vi "Configure.vi"(0 "VISA resource name":refnum<visa-resource-name>, 1 "Voltage(0 Volts)":dbl format="%.3f", 2 "Protection(None:0)":u16(ring) items=["None", "Overcurrent protection", "Overvoltage protection", "Overcurrent and overvoltage protection", "Clear overvoltage condition", "Clear overcurrent protection", "Set time delay"], 5 "Ouput(On:T)":bool=TRUE, 7 "Voltage Mode(F:Immediate)":bool, 9 "Current Mode(F:Immediate)":bool, 11 "error in (no error)":errorcluster, 12 "Current(0 Amps)":dbl format="%.3f", 13 "Overvoltage prot value(50 Volts)":dbl=50.0 format="%.3f", 14 "Time Delay(0 seconds)":dbl format="%.4f") -> (4 "VISA resource name out":refnum<visa-resource-name>, 15 "error out":errorcluster)   [LabVIEW 2012, in "Agilent 66XX Series.lvlib"]
doc: "This vi configures voltage, current, and overvoltage/current protection. It is also responsible for clearing any protection as well as determining whether the output on the power supply changes immediately or is triggered on the HP-IB bus. NOTE: In order to clear the overcurrent or overvoltage condition, the cause of the condition must be removed first. All values are shown in Volts and Amps."
uses:
  <instrlib>/Agilent 66XX Series/Agilent 66XX Series.lvlib
panel:
  # "On"
  # "Off"
  # "Trigger"
  # "Immediate"
  # "Trigger"
  # "Immediate"
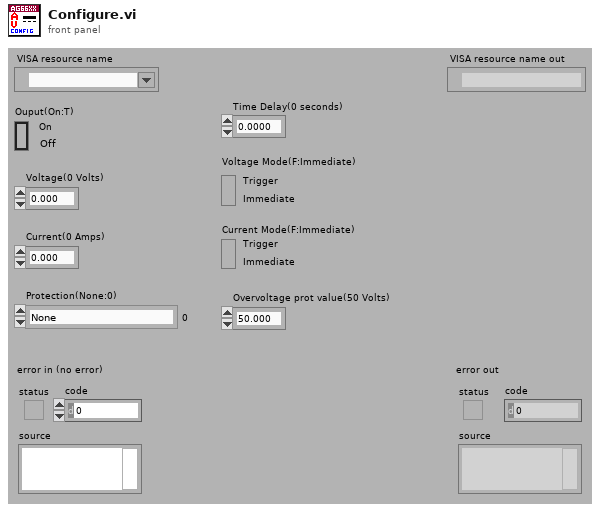
[diagram p1: front panel]
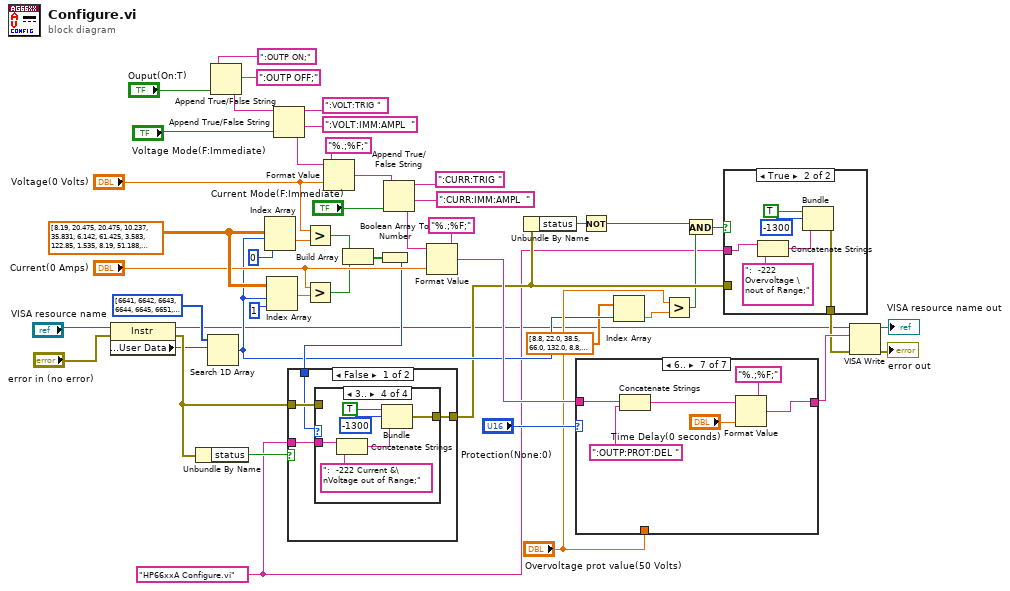
[diagram p0: block diagram]
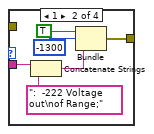
[diagram p4: hidden frame]
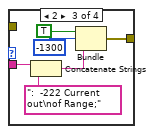
[diagram p5: hidden frame]
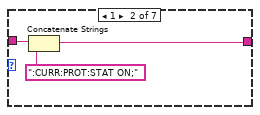
[diagram p8: hidden frame]
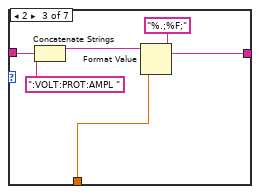
[diagram p9: hidden frame]
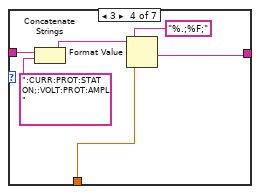
[diagram p10: hidden frame]
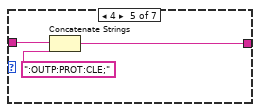
[diagram p11: hidden frame]
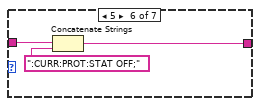
[diagram p12: hidden frame]
diagram:
  w30 = dbl[][] [[8.19, 20.475], [20.475, 10.237], [35.831, 6.142], [61.425, 3.583], [122.85, 1.535], [8.19, 51.188], [20.475, 25.594], [35.831, 15.356], [61.425, 9.214], [122.85, 4.095], [8.19, 225.23], [20.475, 102.37], [35.831, 61.43], [61.425, 35.83], [122.85, 18.43], [5.125, 895.0], [8.19, 592.0], [21.5, 246.0], [32.75, 164.0], [41.0, 131.0], [15.375, 450.0], [30.75, 225.0], [61.5, 112.0], [81.9, 30.71]] ("Range Values")
  w5 = "HP66xxA Configure.vi"
  n1 = property class="Instr"(reference="VISA resource name", error in="error in (no error)") -> (reference out=w4:refnum<visa-resource-name>, error out=w3:errorcluster, "General Settings:User Data"=w2:u32)
  n2 = Unbundle By Name(w3) -> ("status"=w34:bool)
  n3 = Search 1D Array(1D array=u32[] [6641, 6642, 6643, 6644, 6645, 6651, 6652, 6653, 6654, 6655, 6671, 6672, 6673, 6674, 6675, 6680, 6681, 6682, 6683, 6684, 6690, 6691, 6692, 4356] ("Number"), element=w2) -> (index of element=w18:i32)  [unwired: 1 in]
  n4 = Append True/False String(1:"Ouput(On:T)", 2:":OUTP OFF;", 3:":OUTP ON;") -> (0:w11:string)  [unwired: 1 in]
  n5 = Index Array(array=w30, index (row)=w18, index (col)=0) -> (element=w29:dbl)
  n6 = Index Array(array=w30, index (row)=w18, index (col)=1) -> (element=w27:dbl)
  n7 = Append True/False String(1:"Voltage Mode(F:Immediate)", 2:":VOLT:IMM:AMPL  ", 3:":VOLT:TRIG ", 4:w11) -> (0:w47:string)
  n8 = Greater?(x="Voltage(0 Volts)", y=w29) -> (0:w22:bool)
  n9 = Greater?(x="Current(0 Amps)", y=w27) -> (0:w21:bool)
  n10 = Format Value(string ("")=w47, format string="%.;%F;", value (0)="Voltage(0 Volts)") -> (output string=w41:string)
  n11 = Build Array(w22, w21) -> (w20:bool[])
  n12 = Boolean Array To Number(Boolean array=w20) -> (number=w19:u32)
  n13 = case shown="False" w34 {
    tunnel: [w53 w73] -> w10
    tunnel: w3 -> [w52 w73]
    tunnel: w5 -> [w51 _]
    tunnel: w19 -> [w50 _]
    frame False {
      n14 = case shown="3.." w50 {
        tunnel: [w54 w55 w61 w67] -> w53
        tunnel: w52 -> [w54 _ _ _]
        tunnel: w51 -> [_ w56 w62 w68]
        frame ..0 {
        }
        frame 1 {
          n15 = Concatenate Strings(w56, ":  -222 Voltage out\nof Range;") -> (w57:string)
          n16 = Bundle(TRUE, -1300, w57) -> (w55:errorcluster)  [unwired: 1 in]
        }
        frame 2 {
          n17 = Concatenate Strings(w62, ":  -222 Current out\nof Range;") -> (w63:string)
          n18 = Bundle(TRUE, -1300, w63) -> (w61:errorcluster)  [unwired: 1 in]
        }
        frame 3.. {
          n19 = Concatenate Strings(w68, ":  -222 Current &\nVoltage out of Range;") -> (w69:string)
          n20 = Bundle(TRUE, -1300, w69) -> (w67:errorcluster)  [unwired: 1 in]
        }
      }
    }
    frame True {
    }
  }
  n21 = Append True/False String(1:"Current Mode(F:Immediate)", 2:":CURR:IMM:AMPL  ", 3:":CURR:TRIG ", 4:w41) -> (0:w40:string)
  n22 = Format Value(string ("")=w40, format string="%.;%F;", value (0)="Current(0 Amps)") -> (output string=w37:string)
  n23 = Unbundle By Name(w10) -> ("status"=w9:bool)
  n24 = case shown="6.." "Protection(None:0)" {
    tunnel: w37 -> [w74 w77 w83 w86 w92 w94 w101]
    tunnel: [w74 w75 w79 w87 w90 w93 w96] -> w25
    tunnel: "Overvoltage prot value(50 Volts)" -> [_ _ w78 w84 _ _ _]
    frame ..0 {
    }
    frame 1 {
      n25 = Concatenate Strings(w77, ":CURR:PROT:STAT ON;") -> (w75:string)
    }
    frame 2 {
      n26 = Concatenate Strings(w83, ":VOLT:PROT:AMPL ") -> (w81:string)
      n27 = Format Value(string ("")=w81, format string="%.;%F;", value (0)=w78) -> (output string=w79:string)
    }
    frame 3 {
      n28 = Concatenate Strings(w86, ":CURR:PROT:STAT ON;:VOLT:PROT:AMPL ") -> (w89:string)
      n29 = Format Value(string ("")=w89, format string="%.;%F;", value (0)=w84) -> (output string=w87:string)
    }
    frame 4 {
      n30 = Concatenate Strings(w92, ":OUTP:PROT:CLE;") -> (w90:string)
    }
    frame 5 {
      n31 = Concatenate Strings(w94, ":CURR:PROT:STAT OFF;") -> (w93:string)
    }
    frame 6.. {
      n32 = Concatenate Strings(w101, ":OUTP:PROT:DEL ") -> (w98:string)
      n33 = Format Value(string ("")=w98, format string="%.;%F;", value (0)="Time Delay(0 seconds)") -> (output string=w96:string)
    }
  }
  n34 = Not(x=w9) -> (.not. x?=w8:bool)
  n35 = Index Array(array=dbl[] [8.8, 22.0, 38.5, 66.0, 132.0, 8.8, 22.0, 38.5, 66.0, 132.0, 10.0, 24.0, 42.0, 72.0, 144.0, 6.25, 10.0, 25.2, 38.4, 48.0, 18.0, 36.0, 69.0, 96.0] ("Overvoltage values"), index=w18) -> (element=w16:dbl)
  n36 = Greater?(x="Overvoltage prot value(50 Volts)", y=w16) -> (0:w7:bool)
  n37 = And(x=w8, y=w7) -> (x .and. y?=w6:bool)
  n38 = case shown="True" w6 {
    tunnel: w5 -> [_ w104]
    tunnel: w10 -> [w102 _]
    tunnel: [w102 w103] -> w15
    frame False {
    }
    frame True {
      n39 = Concatenate Strings(w104, ":  -222 Overvoltage \nout of Range;") -> (w105:string)
      n40 = Bundle(TRUE, -1300, w105) -> (w103:errorcluster)  [unwired: 1 in]
    }
  }
  n41 = VISA Write(VISA resource name=w4, write buffer=w25, error in (no error)=w15) -> (VISA resource name out=→"VISA resource name out":refnum<visa-resource-name>, error out=→"error out":errorcluster)  [unwired: 1 out]
